vi "Roll.vi"(8 "error in (no error)":errorcluster, 11 "Dice in":refnum<class "Dice.lvclass">) -> (0 "error out":errorcluster, 1 "Stats":cluster{"Max":dbl, "Min":dbl, "Average":dbl}, 2 "Result":dbl, 3 "Dice out":refnum<class "Dice.lvclass">)   [LabVIEW 2021, in "Dice.lvlib" / "Dice.lvclass"]
uses:
  Dice.lvclass
  Dice.lvclass/Dice.ctl
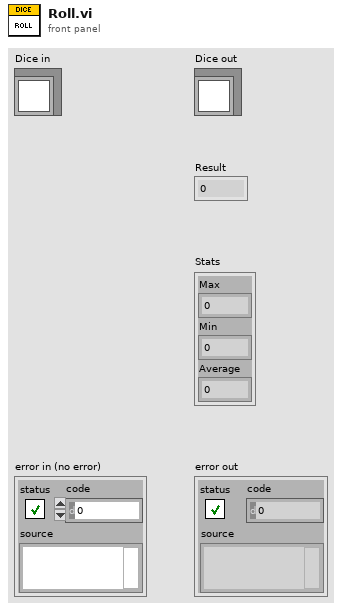
[diagram p1: front panel]
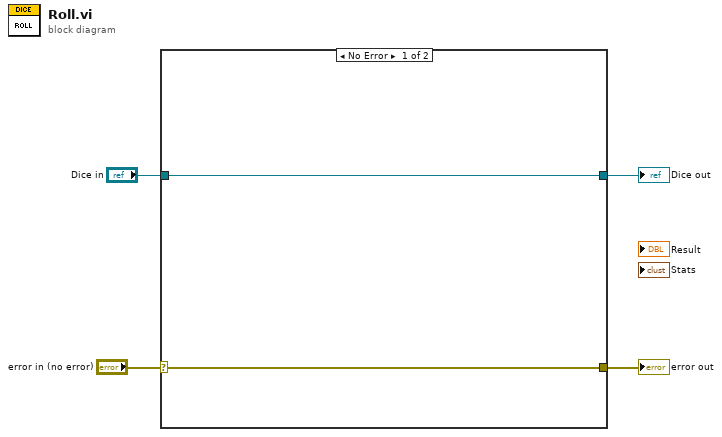
[diagram p0: block diagram]
diagram:
  n1 = case shown="No Error" "error in (no error)" {
    selector: "error in (no error)" -> [w5 w8]
    tunnel: [w5 w8] -> w3
    tunnel: [w6 w7] -> w1
    tunnel: "Dice in" -> [w6 w7]
    frame No Error {
    }
    frame Error {
    }
  }
  "error out" <- w3
  "Dice out" <- w1
